vi "Read Initialization VI Properties.vi"(8 "error in (no error)":errorcluster, 11 "CustomDeviceRepo in":refnum<class "CustomDeviceRepo.lvclass">) -> (0 "error out":errorcluster, 2 "Initialization VI Properties":T1={"Execution"=enum."silent", "Path"={"Path"=path "", "Path Type"=enum."Absolute"}, "Type"=enum."VI", "Position"=enum."centered"}, 3 "CustomDeviceRepo out":refnum<class "CustomDeviceRepo.lvclass">)   [LabVIEW 2015, in "CustomDeviceRepo.lvclass"]
uses:
  CustomDeviceRepo.lvclass
  Custom Device Type Defs/Initialization VI Properties.ctl
  XML Controls/Execution Types.ctl
  XML Controls/Path Cluster.ctl
  CustomDeviceRepo.lvclass/CustomDeviceRepo.ctl
  Configuration Tool.lvlib
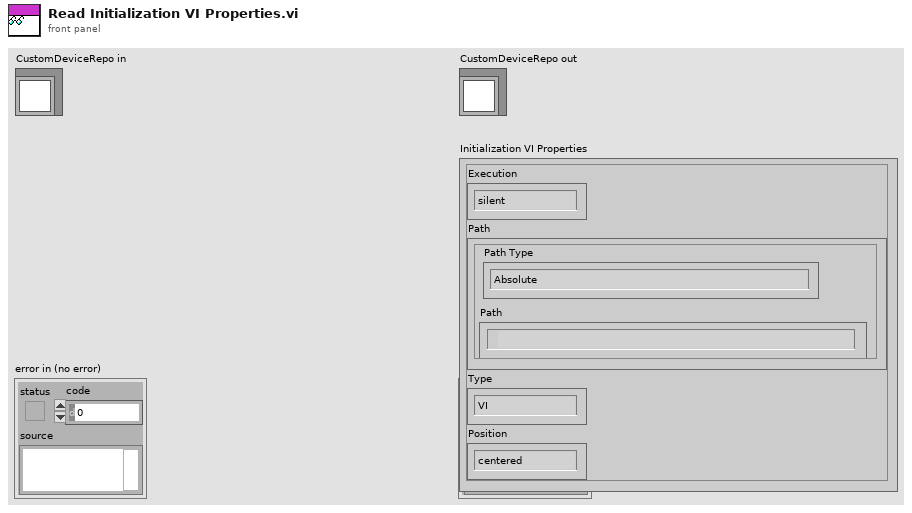
[diagram p1: front panel]
types:
  T1 = typedef "Initialization VI Properties.ctl" = cluster{"Execution":T2, "Path":T3, "Type":enum16{"Action", "VI"}, "Position":enum16{"centered", "mouse pointer"}}
  T2 = typedef "Configuration Tool.lvlib/Execution Types.ctl" = enum16{"silent", "modal", "floating", "default"}
  T3 = typedef "Configuration Tool.lvlib/Path Cluster.ctl" = cluster{"Path":path, "Path Type":enum16{"Absolute", "To Base", "To Common Doc Dir", "To Application Data Dir"}}
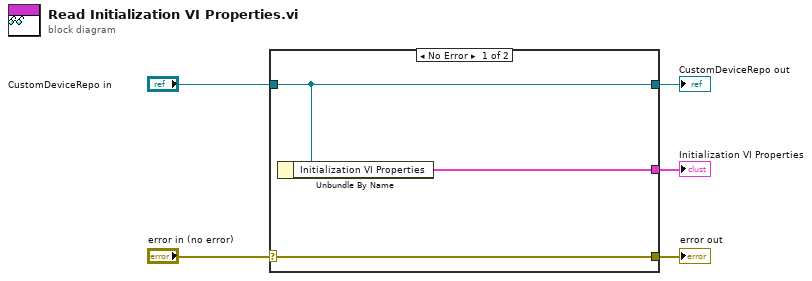
[diagram p0: block diagram]
diagram:
  n1 = case shown="No Error" "error in (no error)" {
    selector: "error in (no error)" -> [w8 w9]
    tunnel: [w8 w9] -> w4
    tunnel: [w7 w10] -> w2
    tunnel: "CustomDeviceRepo in" -> [w7 w10]
    tunnel: [w6 _] -> w1
    frame No Error {
      n2 = Unbundle By Name(w7) -> ("Initialization VI Properties"=w6:T1)
    }
    frame Error {
    }
  }
  "error out" <- w4
  "CustomDeviceRepo out" <- w2
  "Initialization VI Properties" <- w1
